vi "Auto Configuration.vi"() -> ()   [LabVIEW 2017]
uses:
  2018_Trobots_5013_Robot/Support Code/Blocks.ctl
  2018_Trobots_5013_Robot/Support Code/Routines.ctl
  2018_Trobots_5013_Robot/Auto Code/Block Clusters/Far--L.ctl
  2018_Trobots_5013_Robot/Auto Code/Block Clusters/end Sw--sq C1.ctl
  2018_Trobots_5013_Robot/Auto Code/Block Clusters/end cube--C1.ctl
  2018_Trobots_5013_Robot/Auto Code/Block Clusters/C1--d Hi.ctl
  2018_Trobots_5013_Robot/Auto Code/Block Clusters/C1--C3.ctl
  2018_Trobots_5013_Robot/Auto Code/Block Clusters/C3--C4.ctl
  2018_Trobots_5013_Robot/Auto Code/Block Clusters/d Hi--C1.ctl
  2018_Trobots_5013_Robot/Auto Code/Block Clusters/C3--End Sw.ctl
  2018_Trobots_5013_Robot/Auto Code/Block Clusters/C3--cube Sw.ctl
  2018_Trobots_5013_Robot/Auto Code/Block Clusters/M--front RSw.ctl
  2018_Trobots_5013_Robot/Auto Code/Block Clusters/L--C1.ctl
  2018_Trobots_5013_Robot/Auto Code/Block Clusters/C1--end cube.ctl
  2018_Trobots_5013_Robot/Auto Code/Block Clusters/L--end Sw.ctl
  2018_Trobots_5013_Robot/Auto Code/Block Clusters/front Sw--L.ctl
  2018_Trobots_5013_Robot/Auto Code/Block Clusters/M--front LSw.ctl
  2018_Trobots_5013_Robot/Auto Code/Block Clusters/SQ Hi--C1.ctl
  2018_Trobots_5013_Robot/Auto Code/Block Clusters/C1--sq Hi.ctl
  2018_Trobots_5013_Robot/Auto Code/Block Clusters/front Sw--P cube1.ctl
  2018_Trobots_5013_Robot/Auto Code/Block Clusters/P cube1--front Sw.ctl
  Routines and Block Data.ctl
  <vilib>/Rock Robotics/Network Tables/NT Write Boolean.vi
panel:
  out "appended path":path=path "C:/Program Files (x86)/FRC Dashboard/data/C1--end cube.jpg"
  out "Tab Control":T1(tab)=enum."2"
  in  "Far--L":T2={"1a"=0.0, "1d"=100.5, "1s"=0.8}
  in  "L--end Sw":T3={"1d"=48.0, "1s"=0.8, "2t"=3.0, "3a"=90.0, "4d"=21.5, "4s"=0.8}
  in  "end Sw--sq C1":T4={"1a"=-90.0, "1d"=-48.0, "1s"=-0.65, "2d"=67.25, "2s"=0.75}
  in  "end cube--C1":T5={"1a"=124.0, "1d"=0.0, "1s"=0.0, "2a"=0.0}
  in  "C1--d Hi":T6={"1t"=6.5, "2d"=55.0, "2s"=0.65, "3a"=38.0, "4d"=10.0, "4s"=0.5}
  in  "C1--C3":T7={"1a"=90.0, "2d"=185.0, "2s"=1.0}
  in  "C3 to C4":T8
  in  "d Hi--C1":T9={"1a"=38.0, "1d"=18.0, "1s"=0.8, "3t"=0.0, "4d"=33.0, "4s"=1.0}
  in  "C3--End Sw":T10={"1a"=90.0, "1d"=45.31, "1s"=0.8, "2a"=180.0, "3t"=3.0, "4d"=67.25, "4s"=0.7, "5a"=-90.0, "6d"=19.31, "6s"=0.5}
  in  "C3--cube Sw":T11
  in  "M--front LSw":T12={"1d"=14.0, "1s"=1.0, "2a"=-51.5, "3t"=3.0, "4d"=141.0, "4s"=1.0, "5a"=0.0, "6d"=19.5, "6s"=0.5}
  in  "M--front RSw":T13
  in  "front Sw--L":T14={"1d"=14.0, "1s"=-1.0, "2a"=90.0, "3t"=0.0, "4d"=58.25, "4s"=1.0, "5a"=0.0}
  in  "L--C1":T15={"1a"=0.0, "1d"=115.25, "1s"=0.8}
  in  "C1--end cube":T16={"1a"=124.0, "2d"=28.0, "2s"=0.65, "3g"=10.0, "4t"=1.0}
  in  "sq Hi--C1":T17
  in  "C1--sq Hi":T18
  in  "front Sw--P cube1":T19
  in  "P cube1--front Sw":T20={"1a"=0.0, "1d"=40.0, "1s"=-0.85, "2a"=-90.0, "1t"=3.0, "2d"=57.0, "2s"=1.0, "3d"=81.0, "3s"=0.65}
  in  "Remove":bool
  in  "Index":i32=1 min=1 step=1
  in  "Insert":bool
  in  "Routines":T21
  in  "Routine Blocks":T22[](array[typedef])=[enum."M--front LSw", enum."front Sw--L", enum."L--C1", enum."C1--end cube", enum."end cube--C1", enum."C1--d Hi", enum."", enum."", enum."", enum."", enum."", enum."", enum."", enum."", enum."", enum."", enum."", enum."", enum."", enum."", enum."", enum."", enum."", enum."", enum."", enum."", enum.""]
  in  "Cancel":bool
  in  "Done":bool
  in  "Block to Modify":T22=enum."Far--L"
  out "block picture":picture
  # "1"
  # "2"
  # "3"
  # "4"
  # "5"
  # "6"
  # "7"
  # "8"
  # "9"
  # "10"
  # "11"
  # "12"
  # "13"
  # "14"
  # "15"
  # "16"
  # "17"
  # "18"
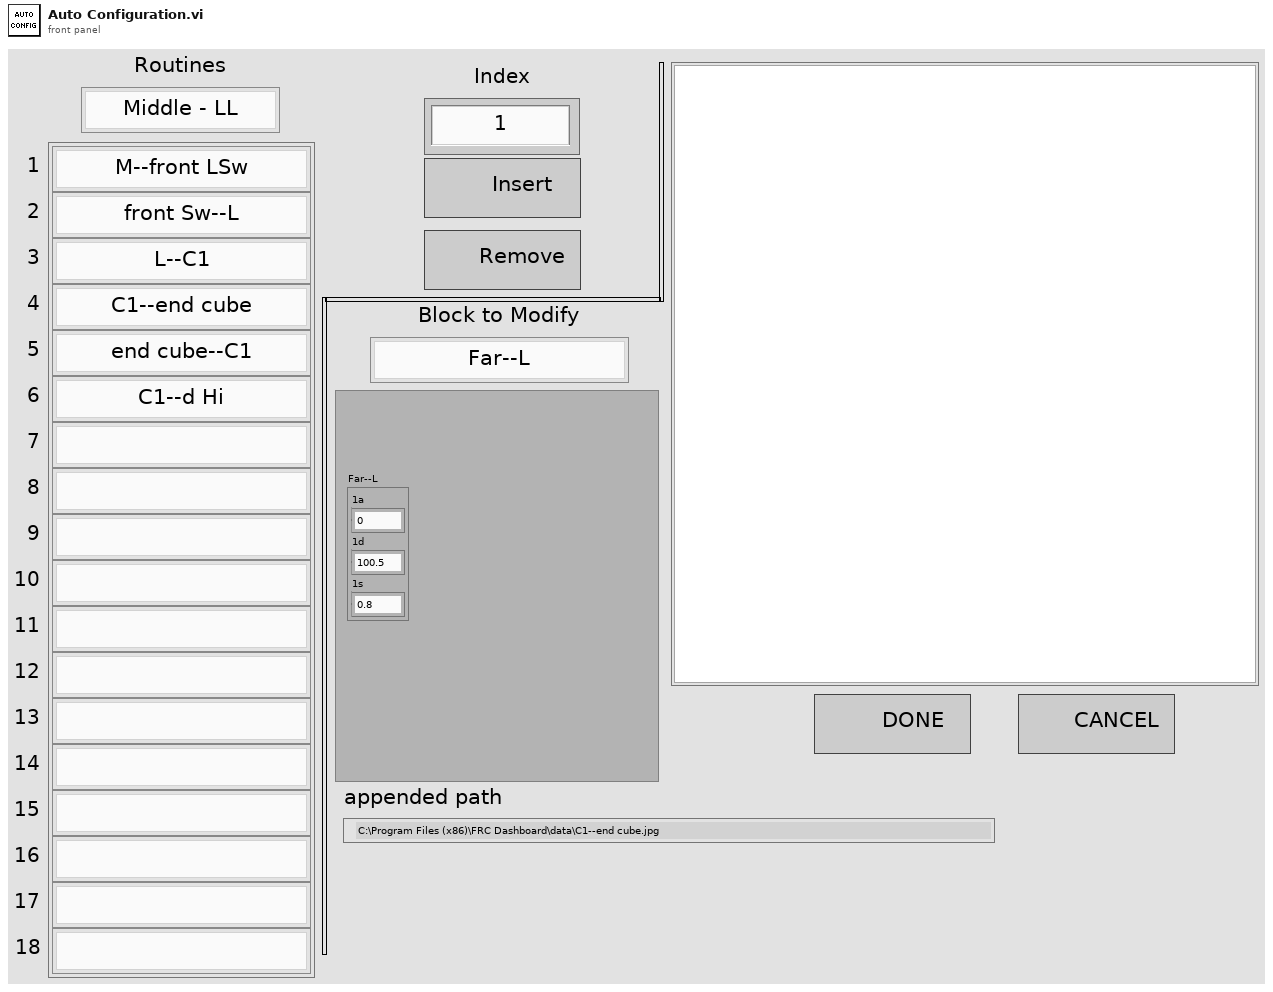
[diagram p1: front panel]
types:
  T1 = enum32{"0", "1", "2", "3", "4", "5", "6", "7", "8", "9", "9 2", "9 3", "9 4", "9 5", "front Sw--L", "L--C1", "C1--end cube", "C1--end cube 2", "C1--end cube 3", "C1--end cube 4", "C1--end cube 5"}
  T2 = typedef "Far--L.ctl" = cluster{"1a":dbl, "1d":dbl, "1s":dbl}
  T3 = typedef "L--end Sw.ctl" = cluster{"1d":dbl, "1s":dbl, "2t":dbl, "3a":dbl, "4d":dbl, "4s":dbl}
  T4 = typedef "end Sw--sq C1.ctl" = cluster{"1a":dbl, "1d":dbl, "1s":dbl, "2d":dbl, "2s":dbl}
  T5 = typedef "end cube--C1.ctl" = cluster{"1a":dbl, "1d":dbl, "1s":dbl, "2a":dbl}
  T6 = typedef "C1--d Hi.ctl" = cluster{"1t":dbl, "2d":dbl, "2s":dbl, "3a":dbl, "4d":dbl, "4s":dbl}
  T7 = typedef "C1--C3.ctl" = cluster{"1a":dbl, "2d":dbl, "2s":dbl}
  T8 = typedef "C3--C4.ctl" = cluster{"1a":dbl, "1d":dbl, "1s":dbl}
  T9 = typedef "d Hi--C1.ctl" = cluster{"1a":dbl, "1d":dbl, "1s":dbl, "3t":dbl, "4d":dbl, "4s":dbl}
  T10 = typedef "C3--End Sw.ctl" = cluster{"1a":dbl, "1d":dbl, "1s":dbl, "2a":dbl, "3t":dbl, "4d":dbl, "4s":dbl, "5a":dbl, "6d":dbl, "6s":dbl}
  T11 = typedef "C3--cube Sw.ctl" = cluster{"1a":dbl, "1d":dbl, "1s":dbl, "2a":dbl, "4d":dbl, "4s":dbl, "5t":dbl}
  T12 = typedef "M--front LSw.ctl" = cluster{"1d":dbl, "1s":dbl, "2a":dbl, "3t":dbl, "4d":dbl, "4s":dbl, "5a":dbl, "6d":dbl, "6s":dbl}
  T13 = typedef "M--front RSw.ctl" = cluster{"1a":dbl, "1d":dbl, "1s":dbl}
  T14 = typedef "front Sw--L.ctl" = cluster{"1d":dbl, "1s":dbl, "2a":dbl, "3t":dbl, "4d":dbl, "4s":dbl, "5a":dbl}
  T15 = typedef "L--C1.ctl" = cluster{"1a":dbl, "1d":dbl, "1s":dbl}
  T16 = typedef "C1--end cube.ctl" = cluster{"1a":dbl, "2d":dbl, "2s":dbl, "3g":dbl, "4t":dbl}
  T17 = typedef "SQ Hi--C1.ctl" = cluster{"1a":dbl, "1d":dbl, "1s":dbl, "2d":dbl, "2s":dbl}
  T18 = typedef "C1--sq Hi.ctl" = cluster{"1d":dbl, "1s":dbl, "2a":dbl, "2d":dbl, "2s":dbl}
  T19 = typedef "front Sw--P cube1.ctl" = cluster{"1a":dbl, "1d":dbl, "1s":dbl, "2a":dbl, "2d":dbl, "2s":dbl, "3d":dbl, "3s":dbl, "1t":dbl}
  T20 = typedef "P cube1--front Sw.ctl" = cluster{"1a":dbl, "1d":dbl, "1s":dbl, "2a":dbl, "1t":dbl, "2d":dbl, "2s":dbl, "3d":dbl, "3s":dbl}
  T21 = typedef "Routines.ctl" = enum16{"Middle - LL", "Middle - LR", "Middle - RL", "Middle - RR", "Far Right - LL", "Far Right - LR", "Far Right - RL", "Far Right - RR", "Far Left - LL", "Far Left - LR", "Far Left - RL", "Far Left - RR"}
  T22 = typedef "Blocks.ctl" = enum16{"", "Wait 1s", "Far--L", "L--end Sw", "end Sw--sq C1", "end cube--C1", "C1--d Hi", "C1--C3", "C3--C4", "d Hi--C1", "C3--end Sw", "C3--cube Sw", "M--front LSw", "M--front RSw", "front Sw--L", "L--C1", "C1--end cube", "sq Hi--C1", "C1--sq Hi", "front Sw--P cube1", "P cube1--front Sw"}
  T23 = typedef "Routines and Block Data.ctl" = cluster{"Routines":T22[][], "Block Data Array":variant[]}
  T24 = typedef "imagedata.ctl" = cluster{"image type":i32, "image depth":i32, "image":u8[], "mask":u8[], "colors":u32[], "Rectangle":cluster{"left":i16, "top":i16, "right":i16, "bottom":i16}}
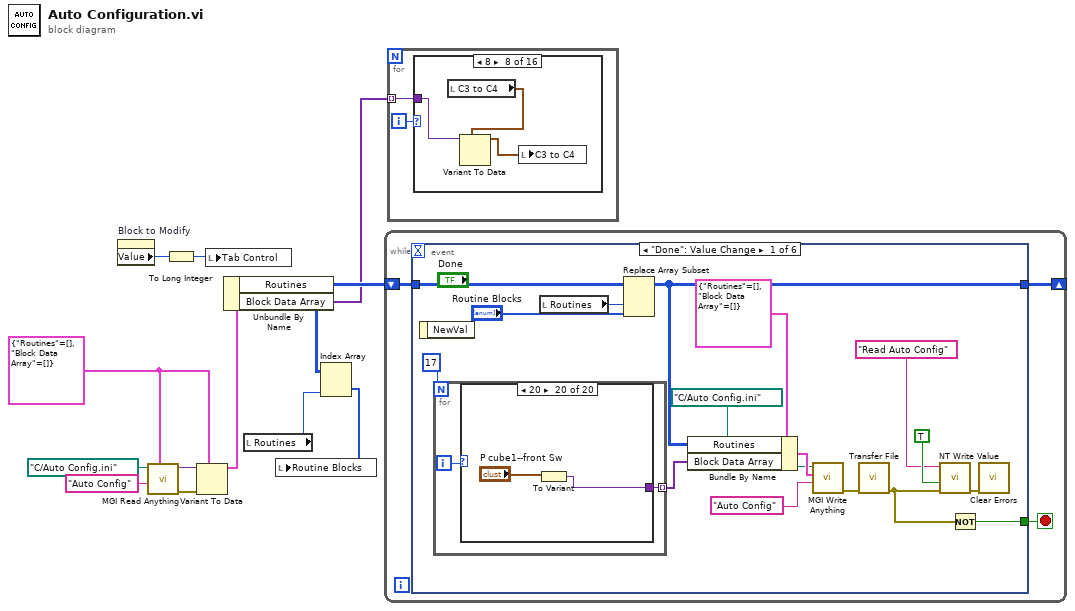
[diagram p0: block diagram]
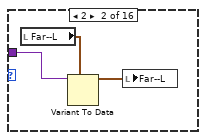
[diagram p3: hidden frame]
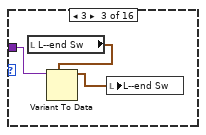
[diagram p4: hidden frame]
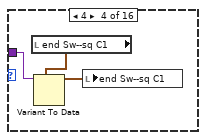
[diagram p5: hidden frame]
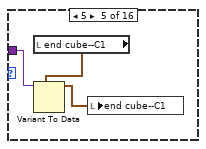
[diagram p6: hidden frame]
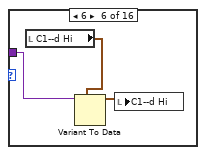
[diagram p7: hidden frame]
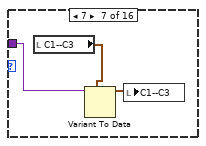
[diagram p8: hidden frame]
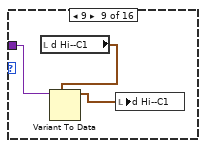
[diagram p9: hidden frame]
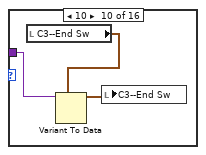
[diagram p10: hidden frame]
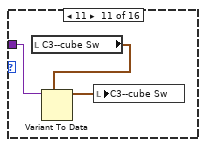
[diagram p11: hidden frame]
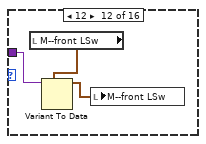
[diagram p12: hidden frame]
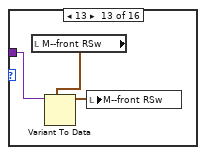
[diagram p13: hidden frame]
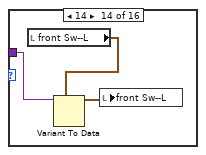
[diagram p14: hidden frame]
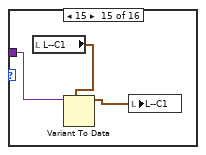
[diagram p15: hidden frame]
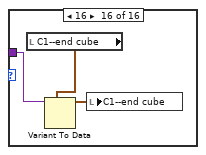
[diagram p16: hidden frame]
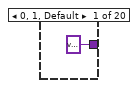
[diagram p17: hidden frame]
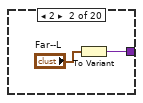
[diagram p18: hidden frame]
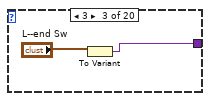
[diagram p19: hidden frame]
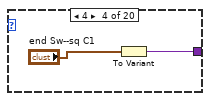
[diagram p20: hidden frame]
diagram:
  w8 = T23 {"Routines"=[], "Block Data Array"=[]} ("Routines and Block Data")
  n1 = property on="Block to Modify" class="Enum (strict)"() -> ("Value"=w3:T22)  [unwired: 2 in, 2 out]
  n2 = call <userlib>:"MGI Read Anything.vi"("Type of Anything"=w8, "Section Name (Name of \"Type of Anything\")"="Auto Config" ("Section Name (Name of \"Type of Anything\")"), "Path (dialog)"=path "C:/Auto Config.ini") -> ("Error Out"=w12:errorcluster, "Anything"=w11:variant)  [unwired: 5 in, 2 out]
  n3 = To Long Integer(number=w3) -> (32bit integer=w2:i32)
  n4 = Variant To Data(error in=w12, type=w8, Variant=w11) -> (data=w9:T23)  [unwired: 1 out]
  n5 = local write "Tab Control"(w2) -> ()
  n6 = Unbundle By Name(w9) -> ("Routines"=w5:T22[][], "Block Data Array"=w1:variant[])
  n7 = local read "Routines"() -> (w6:T21)
  n8 = Index Array(array=w5, index (col)=w6) -> (element=w4:T22[])  [unwired: 1 in]
  n9 = local write "Routine Blocks"(w4) -> ()
  n10 = while {
    shift-right: [w13] -> _
    shift-left: w5 -> [w14]
    stop <- w15 stop-if-true
    n11 = event shown="[0] \"Done\": Value Change" {
      selector: _ -> [_ _ _ _ _ _]
      dyn-events: _ -> [_ _ _ _ _ _]
      timeout: _ -> [_ _ _ _ _ _]
      tunnel: [w16 TRUE _ _ _ _] -> w15
      tunnel: w14 -> [w31 w73 w80 w92 w105 w110]
      tunnel: [w26 w73 w80 w91 w100 w107] -> w13
      event "Done": Value Change {
        n12 = event-data() -> ()  [unwired: 1 in, 1 out]
        n13 = for {
          N: 17 -> [_]
          tunnel: [w33] -> w18 mode=indexing
          i -> [w32]
          n14 = case shown="20" w32 {
            tunnel: [variant ("Variant") w36 w38 w40 w41 w43 w45 w47 w49 w51 w53 w56 w57 w60 w61 w63 w65 w67 w69 w71] -> w33
            frame 0, 1, Default {
            }
            frame 2 {
              n15 = To Variant(anything="Far--L") -> (Variant=w36:variant)
            }
            frame 3 {
              n16 = To Variant(anything="L--end Sw") -> (Variant=w38:variant)
            }
            frame 4 {
              n17 = To Variant(anything="end Sw--sq C1") -> (Variant=w40:variant)
            }
            frame 5 {
              n18 = To Variant(anything="end cube--C1") -> (Variant=w41:variant)
            }
            frame 6 {
              n19 = To Variant(anything="C1--d Hi") -> (Variant=w43:variant)
            }
            frame 7 {
              n20 = To Variant(anything="C1--C3") -> (Variant=w45:variant)
            }
            frame 8 {
              n21 = To Variant(anything="C3 to C4") -> (Variant=w47:variant)
            }
            frame 9 {
              n22 = To Variant(anything="d Hi--C1") -> (Variant=w49:variant)
            }
            frame 10 {
              n23 = To Variant(anything="C3--End Sw") -> (Variant=w51:variant)
            }
            frame 11 {
              n24 = To Variant(anything="C3--cube Sw") -> (Variant=w53:variant)
            }
            frame 12 {
              n25 = To Variant(anything="M--front LSw") -> (Variant=w56:variant)
            }
            frame 13 {
              n26 = To Variant(anything="M--front RSw") -> (Variant=w57:variant)
            }
            frame 14 {
              n27 = To Variant(anything="front Sw--L") -> (Variant=w60:variant)
            }
            frame 15 {
              n28 = To Variant(anything="L--C1") -> (Variant=w61:variant)
            }
            frame 16 {
              n29 = To Variant(anything="C1--end cube") -> (Variant=w63:variant)
            }
            frame 17 {
              n30 = To Variant(anything="sq Hi--C1") -> (Variant=w65:variant)
            }
            frame 18 {
              n31 = To Variant(anything="front Sw--P cube1") -> (Variant=w67:variant)
            }
            frame 19 {
              n32 = To Variant(anything="C1--sq Hi") -> (Variant=w69:variant)
            }
            frame 20 {
              n33 = To Variant(anything="P cube1--front Sw") -> (Variant=w71:variant)
            }
          }
        }
        n34 = local read "Routines"() -> (w21:T21)
        n35 = Replace Array Subset(array=w31, new element="Routine Blocks", index (col)=w21) -> (w26:T22[][])  [unwired: 1 in]
        n36 = Bundle By Name(cluster=T23 {"Routines"=[], "Block Data Array"=[]} ("Routines and Block Data"), "Routines"=w26, "Block Data Array"=w18) -> (w28:T23)
        n37 = call <userlib>:"MGI Write Anything.vi"("Section Name (Name of \"Anything\")"="Auto Config" ("Section Name (Name of \"Anything\")"), "Anything"=w28, "Path (dialog)"=path "C:/Auto Config.ini") -> ("Error Out"=w22:errorcluster)  [unwired: 6 in, 2 out]
        n38 = call "Transfer File.vi"("error in (no error)"=w22) -> ("error out"=w17:errorcluster)  [unwired: 10 in]
        n39 = call-poly <vilib>:"NT Write Value.vi"("error in"=w17, "Boolean"=TRUE, "Name"="Read Auto Config") -> ("error out"=w20:errorcluster)  [unwired: 8 in]
        n40 = Not(x=w17) -> (.not. x?=w16:bool)
        n41 = call <vilib>:"Clear Errors.vi"("error in (no error)"=w20) -> ()  [unwired: 5 in, 2 out]
      }
      event "Cancel": Value Change {
        n42 = event-data() -> ()  [unwired: 1 in, 1 out]
      }
      event Value Change {
        n43 = event-data() -> ()  [unwired: 1 in, 1 out]
        n44 = property on="Block to Modify" class="Enum (strict)"() -> ("Value"=w79:T22)  [unwired: 2 in, 2 out]
        n45 = Format Into String(format string="%s", "Block to Modify") -> (resulting string=w86:string)  [unwired: 2 in, 1 out]
        n46 = To Long Integer(number=w79) -> (32bit integer=→"Tab Control":i32)
        n47 = Concatenate Strings(w86, ".jpg" ("string")) -> (w84:string)
        n48 = Build Path(base path=path "C:/Program Files (x86)/FRC Dashboard/data" ("Path (dialog)"), name or relative path=w84) -> (appended path=w81:path)
        "appended path" <- w81
        n49 = call <vilib>:"Read JPEG File.vi"("path to JPEG file"=w81) -> ("error out"=w76:errorcluster, "image data"=w82:T24)  [unwired: 8 in, 1 out]
        n50 = call <vilib>:"Draw Flattened Pixmap.vi"("image data"=w82) -> ("new picture"=→"block picture":picture)  [unwired: 8 in]
        n51 = call <vilib>:"Clear Errors.vi"("error in (no error)"=w76) -> ()  [unwired: 5 in, 2 out]
      }
      event "Insert": Value Change {
        n52 = event-data() -> ()  [unwired: 1 in, 2 out]
        n53 = local read "Routine Blocks"() -> (w88:T22[])
        n54 = Decrement(x="Index") -> (x-1=w94:i32)
        n55 = local read "Routines"() -> (w90:T21)
        n56 = Insert Into Array(array=w88, index=w94, new element=Blocks."" ("new element/subarray")) -> (w89:T22[])
        n57 = local write "Routine Blocks"(w89) -> ()
        n58 = Replace Array Subset(array=w92, new element=w89, index (col)=w90) -> (w91:T22[][])  [unwired: 1 in]
      }
      event "Remove": Value Change {
        # "take everything below the index in that routine\nand move it all up 1 spot in the array"
        n59 = event-data() -> ()  [unwired: 1 in, 2 out]
        n60 = local read "Index"() -> (w103:i32)
        n61 = local read "Routine Blocks"() -> (w96:T22[])
        n62 = Decrement(x=w103) -> (x-1=w102:i32)
        n63 = Array Subset(array=w96, index=w103) -> (w104:T22[])  [unwired: 1 in]
        n64 = Build Array (concatenate)(w104, Blocks."" ("Blocks")) -> (w99:T22[])
        n65 = local read "Routines"() -> (w101:T21)
        n66 = Replace Array Subset(array=w96, new element=w99, index=w102) -> (w97:T22[])
        n67 = Replace Array Subset(array=w105, new element=w97, index (col)=w101) -> (w100:T22[][])  [unwired: 1 in]
        n68 = local write "Routine Blocks"(w97) -> ()
      }
      event Value Change {
        n69 = event-data() -> ("OldVal"=w108:T21)  [unwired: 1 in]
        n70 = local read "Routine Blocks"() -> (w109:T22[])
        n71 = Replace Array Subset(array=w110, new element=w109, index (col)=w108) -> (w107:T22[][])  [unwired: 1 in]
        n72 = Index Array(array=w107, index (col)="Routines") -> (element=w111:T22[])  [unwired: 1 in]
        n73 = local write "Routine Blocks"(w111) -> ()
      }
    }
  }
  n74 = for {
    tunnel: w1 -> [w112] mode=indexing
    i -> [w113]
    n75 = case shown="8" w113 {
      tunnel: w112 -> [_ w116 w119 w122 w125 w126 w129 w134 w137 w138 w141 w146 w148 w150 w155 w157]
      frame 0, Default {
      }
      frame 2 {
        n76 = local read "Far--L"() -> (w115:T2)
        n77 = Variant To Data(type=w115, Variant=w116) -> (data=w114:T2)  [unwired: 1 in, 1 out]
        n78 = local write "Far--L"(w114) -> ()
      }
      frame 3 {
        n79 = local read "L--end Sw"() -> (w118:T3)
        n80 = Variant To Data(type=w118, Variant=w119) -> (data=w117:T3)  [unwired: 1 in, 1 out]
        n81 = local write "L--end Sw"(w117) -> ()
      }
      frame 4 {
        n82 = local read "end Sw--sq C1"() -> (w121:T4)
        n83 = Variant To Data(type=w121, Variant=w122) -> (data=w120:T4)  [unwired: 1 in, 1 out]
        n84 = local write "end Sw--sq C1"(w120) -> ()
      }
      frame 5 {
        n85 = local read "end cube--C1"() -> (w124:T5)
        n86 = Variant To Data(type=w124, Variant=w125) -> (data=w123:T5)  [unwired: 1 in, 1 out]
        n87 = local write "end cube--C1"(w123) -> ()
      }
      frame 6 {
        n88 = local read "C1--d Hi"() -> (w127:T6)
        n89 = Variant To Data(type=w127, Variant=w126) -> (data=w128:T6)  [unwired: 1 in, 1 out]
        n90 = local write "C1--d Hi"(w128) -> ()
      }
      frame 7 {
        n91 = local read "C1--C3"() -> (w130:T7)
        n92 = Variant To Data(type=w130, Variant=w129) -> (data=w131:T7)  [unwired: 1 in, 1 out]
        n93 = local write "C1--C3"(w131) -> ()
      }
      frame 8 {
        n94 = local read "C3 to C4"() -> (w133:T8)
        n95 = Variant To Data(type=w133, Variant=w134) -> (data=w132:T8)  [unwired: 1 in, 1 out]
        n96 = local write "C3 to C4"(w132) -> ()
      }
      frame 9 {
        n97 = local read "d Hi--C1"() -> (w136:T9)
        n98 = Variant To Data(type=w136, Variant=w137) -> (data=w135:T9)  [unwired: 1 in, 1 out]
        n99 = local write "d Hi--C1"(w135) -> ()
      }
      frame 10 {
        n100 = local read "C3--End Sw"() -> (w140:T10)
        n101 = Variant To Data(type=w140, Variant=w138) -> (data=w139:T10)  [unwired: 1 in, 1 out]
        n102 = local write "C3--End Sw"(w139) -> ()
      }
      frame 11 {
        n103 = local read "C3--cube Sw"() -> (w142:T11)
        n104 = Variant To Data(type=w142, Variant=w141) -> (data=w143:T11)  [unwired: 1 in, 1 out]
        n105 = local write "C3--cube Sw"(w143) -> ()
      }
      frame 12 {
        n106 = local read "M--front LSw"() -> (w145:T12)
        n107 = Variant To Data(type=w145, Variant=w146) -> (data=w144:T12)  [unwired: 1 in, 1 out]
        n108 = local write "M--front LSw"(w144) -> ()
      }
      frame 13 {
        n109 = local read "M--front RSw"() -> (w147:T13)
        n110 = Variant To Data(type=w147, Variant=w148) -> (data=w149:T13)  [unwired: 1 in, 1 out]
        n111 = local write "M--front RSw"(w149) -> ()
      }
      frame 14 {
        n112 = local read "front Sw--L"() -> (w151:T14)
        n113 = Variant To Data(type=w151, Variant=w150) -> (data=w152:T14)  [unwired: 1 in, 1 out]
        n114 = local write "front Sw--L"(w152) -> ()
      }
      frame 15 {
        n115 = local read "L--C1"() -> (w154:T15)
        n116 = Variant To Data(type=w154, Variant=w155) -> (data=w153:T15)  [unwired: 1 in, 1 out]
        n117 = local write "L--C1"(w153) -> ()
      }
      frame 16 {
        n118 = local read "C1--end cube"() -> (w156:T16)
        n119 = Variant To Data(type=w156, Variant=w157) -> (data=w158:T16)  [unwired: 1 in, 1 out]
        n120 = local write "C1--end cube"(w158) -> ()
      }
    }
  }
